vi "Parse PROCAR.vi"(10 "Extract Decomposed Band?":bool, 11 "Path":path) -> (0 "KS Bandgap (eV)":dbl, 1 "CBM Band Index":i32, 2 "Decomposed Band Structure":T1(array[cluster]), 3 "Band Structure":T2(array[cluster]))   [LabVIEW 2010]
uses:
  <vilib>/Utility/error.llb/DialogType.ctl
  <vilib>/Analysis/_algsub.llb/Real Vector Norm.vi
  <vilib>/Analysis/NI_AALPro.lvlib
panel:
  out "CBM (eV)":dbl
  out "VBM (eV)":dbl
  in  "balance parameter":dbl=-1.0
  in  "# of points per slope":i16=4
  out "System XY Graph 3":cluster{i32[], "dY/dX":dbl[]}[](graph)
  out "1st Deriv":cluster{i32[], "Best Cubic Spline Fit":dbl[]}[](graph)
  out "Calc time (ms)":u32
  in  "Bands to Plot":i32[](array[numeric])
  out "System XY Graph":cluster{i32[], dbl[]}[](graph)
  out "# of Ions":i32
  out "# of Bands":i32
  out "# k points":i32
  # "Gamma"
  # "X"
  # "L"
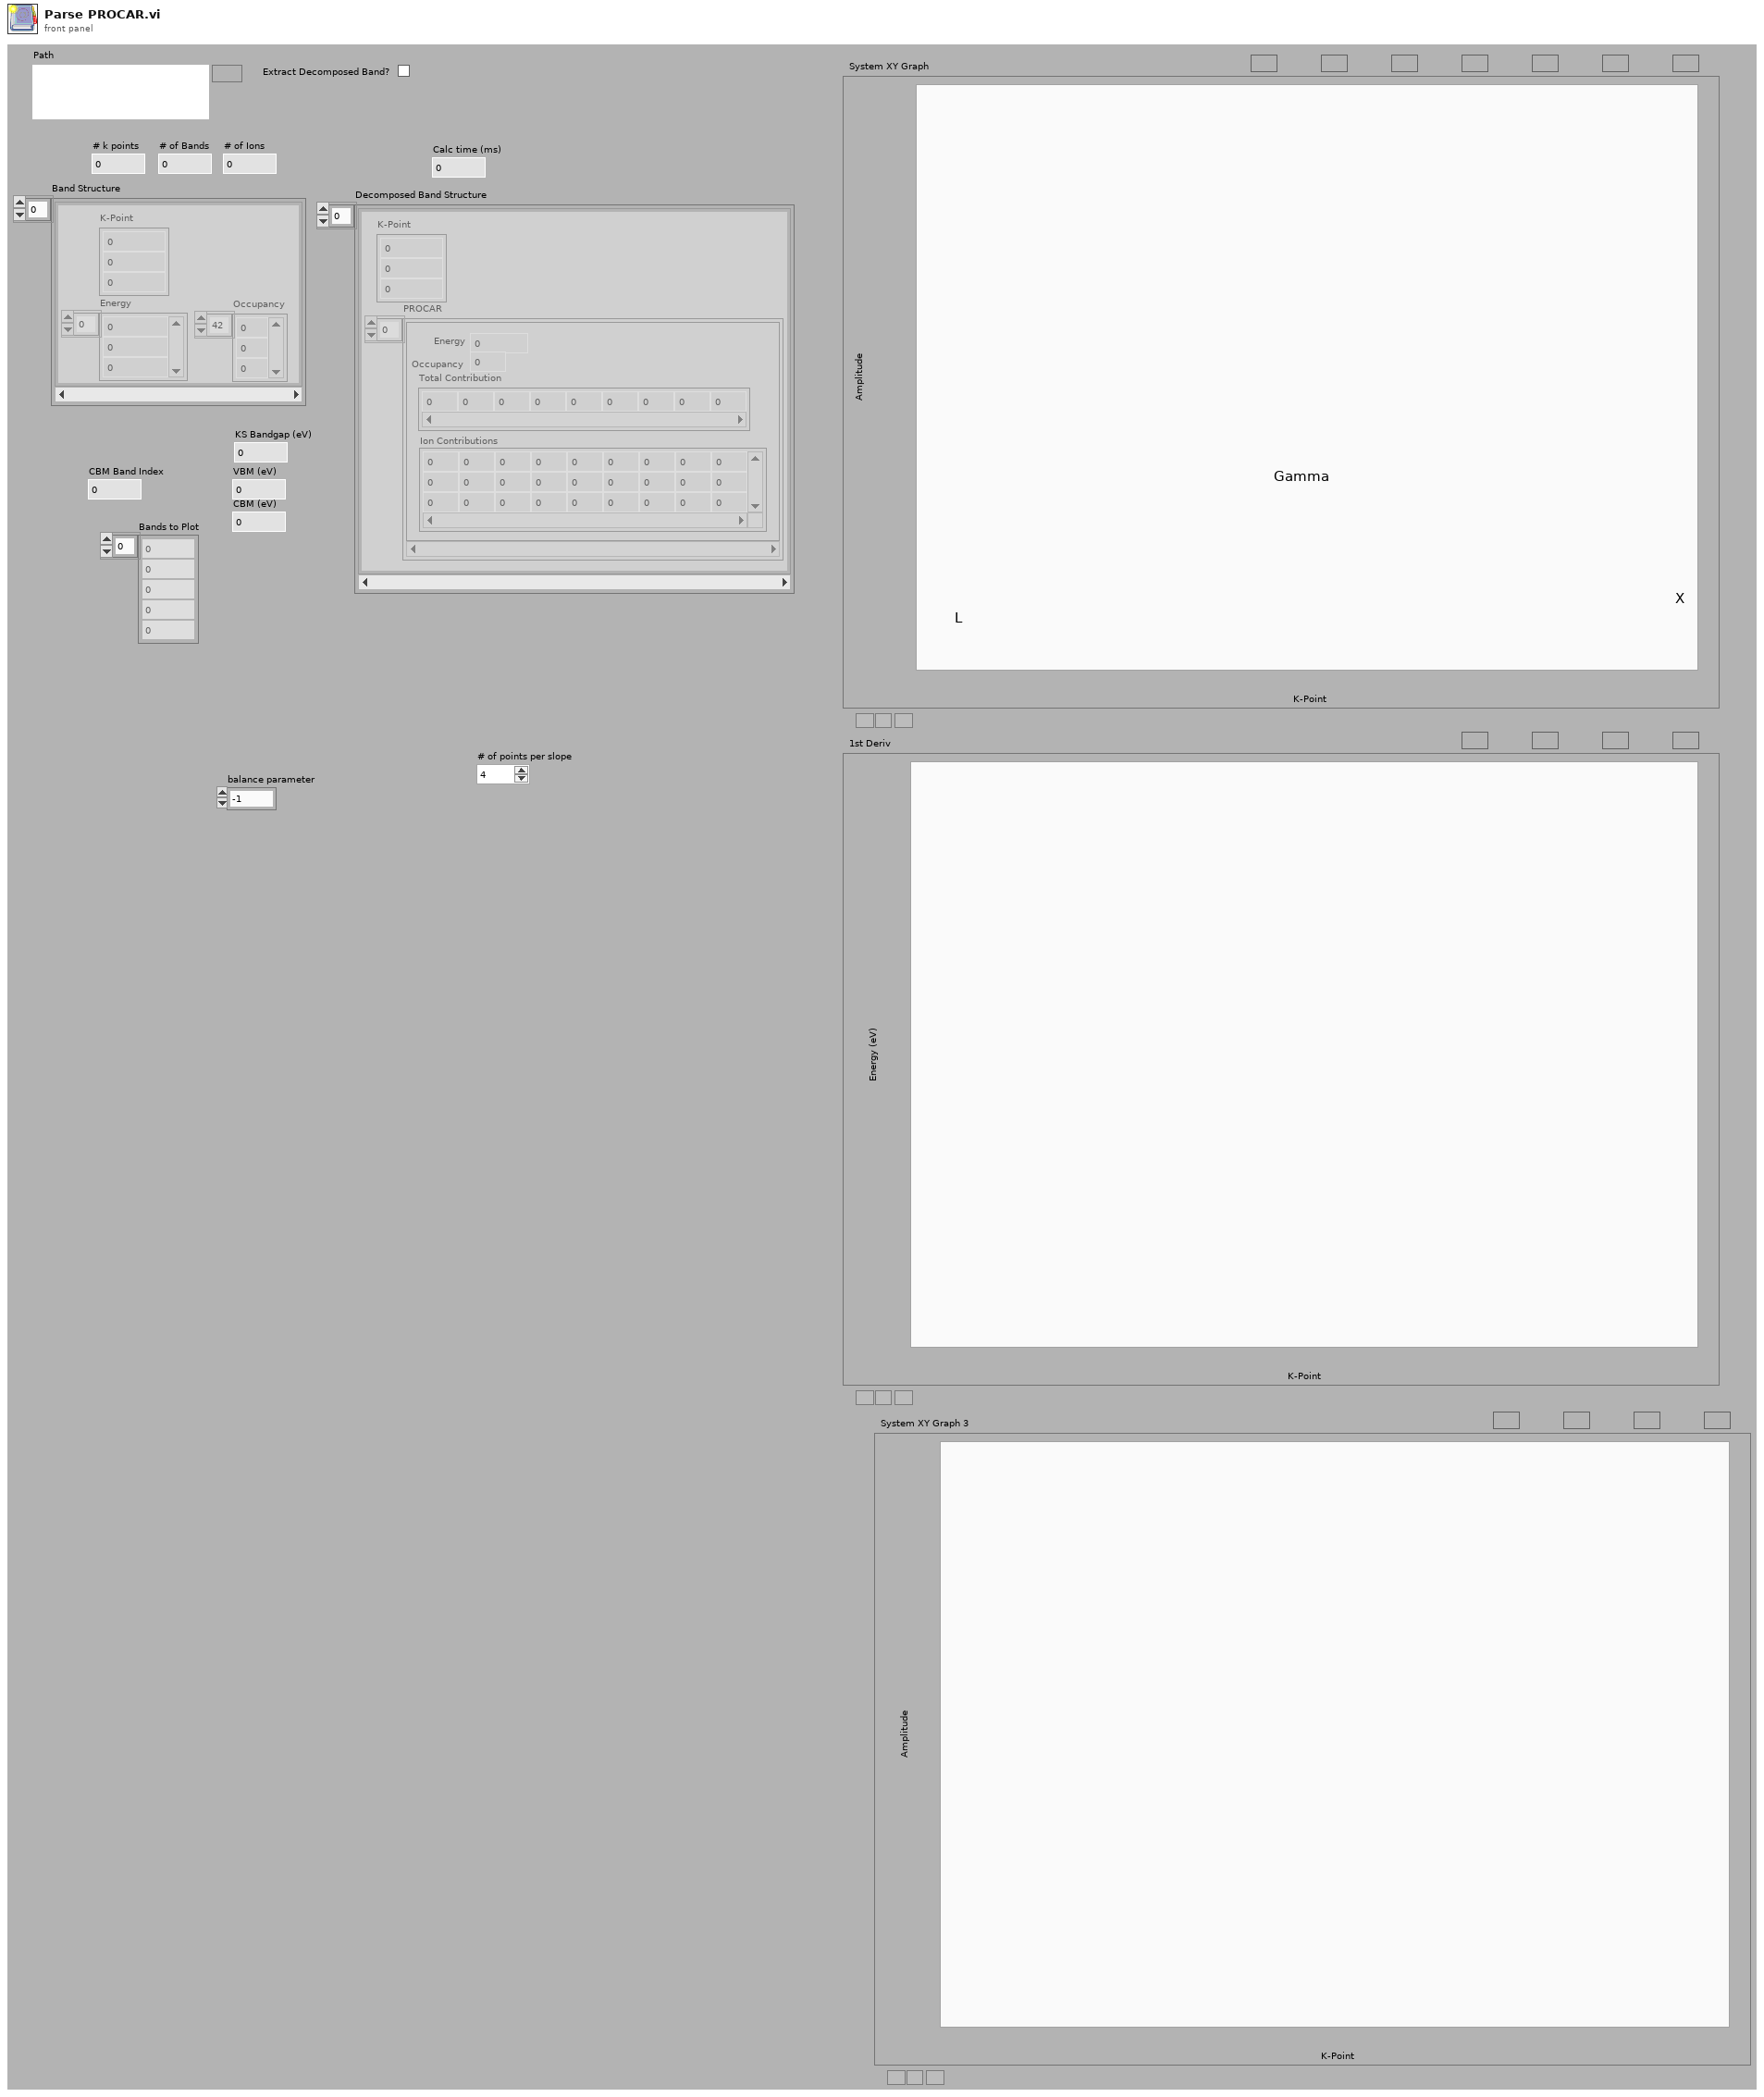
[diagram p1: front panel]
types:
  T1 = cluster{"K-Point":dbl[], "PROCAR":cluster{"Energy":dbl, "Occupancy":dbl, "Total Contribution":dbl[], "Ion Contributions":dbl[][]}[]}[]
  T2 = cluster{"K-Point":dbl[], "Energy":dbl[], "Occupancy":dbl[]}[]
  T3 = cluster{"number 3":dbl[], cluster{dbl, dbl, dbl[], dbl[][]}[]}[]
  T4 = cluster{"number 3":dbl[], "number 3":dbl[], "number 3":dbl[]}
  T5 = cluster{"number 3":dbl[], cluster{dbl, dbl, dbl[], dbl[][]}[]}
  T6 = cluster{"number 3":dbl[], "number 3":dbl[], "number 3":dbl[]}[]
  T7 = typedef "DialogType.ctl" = u16
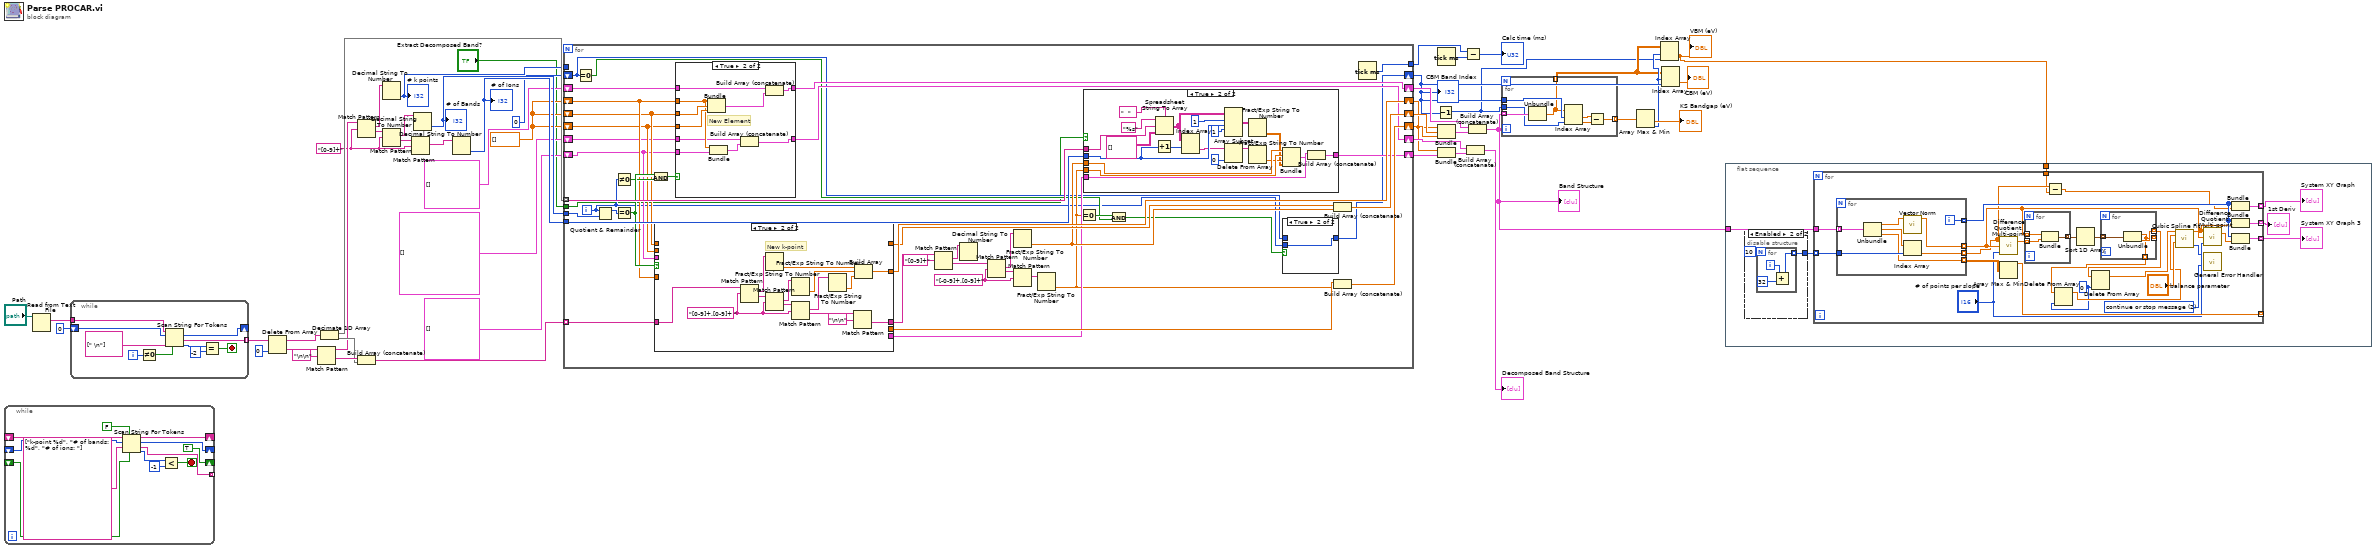
[diagram p0: block diagram]
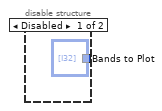
[diagram p2: hidden frame]
diagram:
  w27 = dbl[] [] ("number 3")
  w34 = "[0-9]+"
  n1 = while {
    shift-right: [w59] -> _
    shift-left: _ -> [w60]
    tunnel: [w58] -> _ mode=indexing
    shift-right: [w57] -> _
    shift-left: _ -> [w56]
    shift-right: [TRUE ("allow empty tokens? (F)")] -> _
    shift-left: _ -> [w52]
    stop <- w53 stop-if-true
    n2 = Scan String For Tokens(4:w52, 5:FALSE ("allow empty tokens? (F)"), 7:string[] ["k-point %d", "# of bands: %d", "# of ions: "] ("operators (none)"), 8:w56, 9:w60) -> (0:w55:i32, 1:w58:string, 2:w57:i32, 3:w59:string)  [unwired: 1 in]
    n3 = Less?(x=w55, y=-1) -> (x < y?=w53:bool)
  }
  n4 = Read from Text File(file (use dialog)="Path") -> (text=w48:string)  [unwired: 3 in, 3 out]
  n5 = while {
    tunnel: w48 -> [w71]
    shift-right: [w63] -> _
    shift-left: 0 ("offset past token") -> [w62]
    tunnel: [w70] -> w46 mode=indexing
    i -> [w68]
    stop <- w64 stop-if-true
    n6 = Not Equal To 0?(x=w68) -> (x != 0?=w67:bool)
    n7 = Scan String For Tokens(4:w67, 6:string[] [" \n"] ("delimiters (\\s,\\t,\\r,\\n)"), 8:w62, 9:w71) -> (0:w66:i32, 1:w70:string, 2:w63:i32)  [unwired: 2 in, 1 out]
    n8 = Equal?(x=w66, y=-2) -> (x = y?=w64:bool)
  }
  n9 = Delete From Array(array=w46, index=0) -> (deleted portion=w44:string, array with subset deleted=w45:string[])  [unwired: 1 in]
  n10 = Match Pattern(string=w44, regular expression="\n\n") -> (before substring=w37:string, after substring=w42:string)  [unwired: 1 in, 2 out]
  n11 = Decimate 1D Array(w45) -> (w38:string[], w41:string[])
  n12 = Match Pattern(string=w37, regular expression=w34) -> (match substring=w33:string, after substring=w36:string)  [unwired: 1 in, 2 out]
  n13 = Build Array (concatenate)(w42, w41) -> (w39:string[])
  n14 = Decimal String To Number(string=w33) -> (number=w26:i32)  [unwired: 2 in, 1 out]
  "# k points" <- w26
  n15 = Match Pattern(string=w36, regular expression=w34) -> (match substring=w32:string, after substring=w35:string)  [unwired: 1 in, 2 out]
  n16 = Match Pattern(string=w35, regular expression=w34) -> (match substring=w31:string)  [unwired: 1 in, 3 out]
  n17 = Decimal String To Number(string=w32) -> (number=w29:i32)  [unwired: 2 in, 1 out]
  "# of Bands" <- w29
  n18 = Decimal String To Number(string=w31) -> (number=w30:i32)  [unwired: 2 in, 1 out]
  "# of Ions" <- w30
  n19 = for {
    tunnel: w38 -> [w112] mode=indexing
    tunnel: w39 -> [w103] mode=indexing
    tunnel: w30 -> [w111]
    tunnel: w29 -> [w93]
    shift-right: [w104] -> w18
    shift-left: w27 -> [w92]
    shift-right: [w88] -> w23
    shift-left: T2 [] ("Band Structure") -> [w89]
    shift-right: [w98] -> w25
    shift-left: w27 -> [w91]
    shift-right: [w99] -> w24
    shift-left: w27 -> [w90]
    tunnel: w26 -> [_]
    shift-right: [w85] -> w17
    shift-left: cluster{dbl, dbl, dbl[], dbl[][]}[] [] -> [w82]
    shift-right: [w84] -> w19
    shift-left: T3 [] -> [w83]
    shift-right: [w76] -> w6
    shift-left: 0 ("# of Ions 2") -> [w74]
    tunnel: [w73] -> w8
    tunnel: "Extract Decomposed Band?" -> [w72]
    i -> [w75]
    w105 = "[-0-9]+.[0-9]+" ("regular expression")
    n20 = Equal To 0?(x=w74) -> (x = 0?=w78:bool)
    n21 = Quotient & Remainder(x=w75, y=w93) -> (x-y*floor(x/y)=w102:i32)  [unwired: 1 out]
    n22 = Not Equal To 0?(x=w75) -> (x != 0?=w94:bool)
    n23 = Equal To 0?(x=w102) -> (x = 0?=w95:bool)
    n24 = And(x=w95, y=w94) -> (x .and. y?=w87:bool)
    n25 = case shown="True" w95 {
      tunnel: w103 -> [w151 w165]
      tunnel: w92 -> [w150 _]
      tunnel: [w150 w152] -> w104
      tunnel: [w151 w164] -> w106
      tunnel: w91 -> [w149 _]
      tunnel: w90 -> [w148 _]
      tunnel: [w149 _] -> w97
      tunnel: [w148 _] -> w96
      tunnel: w82 -> [w147 _]
      tunnel: [w147 _] -> w81
      frame False {
        # "Only new band"
      }
      frame True {
        w161 = "[0-9]+.[0-9]+ " ("regular expression")
        # "New k-point"
        n26 = Match Pattern(string=w165, regular expression=w161) -> (match substring=w155:string, after substring=w163:string)  [unwired: 1 in, 2 out]
        n27 = Fract/Exp String To Number(string=w155) -> (number=w159:dbl)  [unwired: 3 in, 1 out]
        n28 = Match Pattern(string=w163, regular expression=w161) -> (match substring=w160:string, after substring=w162:string)  [unwired: 1 in, 2 out]
        n29 = Fract/Exp String To Number(string=w160) -> (number=w158:dbl)  [unwired: 3 in, 1 out]
        n30 = Match Pattern(string=w162, regular expression=w161) -> (match substring=w156:string, after substring=w154:string)  [unwired: 1 in, 2 out]
        n31 = Fract/Exp String To Number(string=w156) -> (number=w157:dbl)  [unwired: 3 in, 1 out]
        n32 = Match Pattern(string=w154, regular expression="\n\n") -> (after substring=w164:string)  [unwired: 1 in, 3 out]
        n33 = Build Array(w159, w158, w157) -> (w152:dbl[])
      }
    }
    n34 = case shown="True" w87 {
      tunnel: w92 -> [_ w141]
      tunnel: w91 -> [_ w146]
      tunnel: w90 -> [_ w145]
      tunnel: w89 -> [w136 w144]
      tunnel: [w136 w143] -> w88
      tunnel: w82 -> [_ w142]
      tunnel: [w135 w139] -> w84
      tunnel: w83 -> [w135 w138]
      frame False {
      }
      frame True {
        # "New Element"
        n35 = Bundle("number 3"=w141, "number 3"=w146, "number 3"=w145) -> (w137:T4)  [unwired: 1 in]
        n36 = Bundle("number 3"=w141, w142) -> (w140:T5)  [unwired: 1 in]
        n37 = Build Array (concatenate)(w138, w140) -> (w139:T3)
        n38 = Build Array (concatenate)(w144, w137) -> (w143:T6)
      }
    }
    n39 = Match Pattern(string=w106, regular expression="[0-9]+") -> (match substring=w107:string, after substring=w110:string)  [unwired: 1 in, 2 out]
    n40 = Decimal String To Number(string=w107) -> ()  [unwired: 2 in, 2 out]
    n41 = Match Pattern(string=w110, regular expression=w105) -> (match substring=w101:string, after substring=w109:string)  [unwired: 1 in, 2 out]
    n42 = Fract/Exp String To Number(string=w101) -> (number=w86:dbl)  [unwired: 3 in, 1 out]
    n43 = Match Pattern(string=w109, regular expression=w105) -> (match substring=w100:string)  [unwired: 1 in, 3 out]
    n44 = Fract/Exp String To Number(string=w100) -> (number=w80:dbl)  [unwired: 3 in, 1 out]
    n45 = Equal To 0?(x=w80) -> (x = 0?=w79:bool)
    n46 = case shown="True" w72 {
      tunnel: w112 -> [_ w132]
      tunnel: w111 -> [_ w131]
      tunnel: w86 -> [_ w130]
      tunnel: [_ w129] -> w85
      tunnel: w81 -> [_ w128]
      tunnel: w80 -> [_ w127]
      frame False {
      }
      frame True {
        n47 = Increment(x=w131) -> (x+1=w119:i32)
        n48 = Spreadsheet String To Array(delimiter (Tab)="  ", format string="%s", spreadsheet string=w132, array type (2D Dbl)=string[][] []) -> (array=w120:string[][])
        n49 = Index Array(array=w120, index (row)=w119) -> (element=w118:string[])  [unwired: 1 in]
        n50 = Array Subset(array=w120, index (row)=1 ("index"), length (row)=w131, index (col)=1 ("index")) -> (w115:string[][])  [unwired: 1 in]
        n51 = Delete From Array(array=w118, index=0) -> (array with subset deleted=w116:string[])  [unwired: 1 in, 1 out]
        n52 = Fract/Exp String To Number(string=w115) -> (number=w113:dbl[][])  [unwired: 3 in, 1 out]
        n53 = Fract/Exp String To Number(string=w116) -> (number=w114:dbl[])  [unwired: 3 in, 1 out]
        n54 = Bundle(w130, w127, w114, w113) -> (w126:cluster{dbl, dbl, dbl[], dbl[][]})  [unwired: 1 in]
        n55 = Build Array (concatenate)(w128, w126) -> (w129:cluster{dbl, dbl, dbl[], dbl[][]}[])
      }
    }
    n56 = And(x=w79, y=w78) -> (x .and. y?=w77:bool)
    n57 = case shown="True" w77 {
      tunnel: [w133 w134] -> w76
      tunnel: w75 -> [_ w134]
      tunnel: w74 -> [w133 _]
      frame False {
      }
      frame True {
      }
    }
    n58 = Build Array (concatenate)(w97, w86) -> (w98:dbl[])
    n59 = Build Array (concatenate)(w96, w80) -> (w99:dbl[])
    n60 = Tick Count (ms)() -> (millisecond timer value=w73:u32)
  }
  "CBM Band Index" <- w6
  n61 = Decrement(x=w6) -> (x-1=w3:i32)
  n62 = Tick Count (ms)() -> (millisecond timer value=w12:u32)
  n63 = Bundle("number 3"=w18, "number 3"=w25, "number 3"=w24) -> (w22:T4)  [unwired: 1 in]
  n64 = Bundle("number 3"=w18, w17) -> (w16:T5)  [unwired: 1 in]
  n65 = Subtract(x=w8, y=w12) -> (x-y=→"Calc time (ms)":u32)
  n66 = Build Array (concatenate)(w19, w16) -> (→"Decomposed Band Structure":T3)
  n67 = Build Array (concatenate)(w23, w22) -> (w13:T6)
  "Band Structure" <- w13
  n68 = for {
    tunnel: w13 -> [w172] mode=indexing
    tunnel: w3 -> [w170]
    tunnel: w6 -> [w171]
    tunnel: [w167] -> w10 mode=indexing
    tunnel: [w166] -> w4 mode=indexing
    n69 = Unbundle(w172) -> ("number 3"=w166:dbl[])  [unwired: 2 out]
    n70 = Index Array(array=w166, index #1=w171, index #2=w170) -> (element #1=w169:dbl, element #2=w168:dbl)
    n71 = Subtract(x=w169, y=w168) -> (x-y=w167:dbl)
  }
  n72 = Array Max & Min(array=w10) -> (min value=→"KS Bandgap (eV)":dbl, min index (indices)=w5:i32)  [unwired: 2 out]
  n73 = Index Array(array=w4, index (row)=w5, index (col)=w3) -> (element=w1:dbl)
  "VBM (eV)" <- w1
  n74 = Index Array(array=w4, index (row)=w5, index (col)=w6) -> (element=→"CBM (eV)":dbl)
  n75 = flat-sequence {
    tunnel: w13 -> [w178]
    tunnel: w1 -> [w173]
    frame #0 {
      n76 = disable-structure shown="Enabled" {
        disable-tunnel: ["Bands to Plot" w181] -> w177
        frame Disabled {
        }
        frame Enabled {
          n77 = for {
            N: 10 -> [_]
            tunnel: [w183] -> w181 mode=indexing
            i -> [w184]
            n78 = Add(x=w184, y=32) -> (x+y=w183:i32)
          }
        }
      }
      n79 = for {
        tunnel: w178 -> [w209]
        tunnel: w177 -> [w210] mode=indexing
        tunnel: [w208] -> w176 mode=indexing
        tunnel: [w206] -> _ mode=indexing
        tunnel: [w205] -> w175 mode=indexing
        tunnel: [w203] -> w174 mode=indexing
        tunnel: w173 -> [w186]
        w188 = 0 ("index")
        w193 = T7 2 items=["no dialog", "OK message", "continue or stop message", "OK message + warnings", "continue/stop + warnings"] ("type of dialog (OK msg:1)")
        n80 = for {
          tunnel: w210 -> [w222]
          tunnel: w209 -> [w224] mode=indexing
          tunnel: [w221] -> w187 mode=indexing
          tunnel: [w220] -> w201 mode=indexing
          tunnel: [w219] -> w207 mode=indexing
          tunnel: [w217] -> w197 mode=indexing
          i -> [w220]
          n81 = Unbundle(w224) -> ("number 3"=w218:dbl[], "number 3"=w223:dbl[], "number 3"=w219:dbl[])
          n82 = call-poly <vilib>:"Vector Norm.vi"("Input Vector"=w218) -> ("norm"=w217:dbl)  [unwired: 9 in, 1 out]
          n83 = Index Array(array=w223, index=w222) -> (element=w221:dbl)
        }
        n84 = call "Difference Quotient, Multi-point.vi"("# of points per slope"="# of points per slope", "X"=w197, "Y"=w187) -> ("dY/dX"=w200:dbl[])  [unwired: 1 in]
        n85 = Array Max & Min(array=w207) -> (max value=w206:dbl)  [unwired: 3 out]
        n86 = for {
          tunnel: w197 -> [w215] mode=indexing
          tunnel: w200 -> [w216] mode=indexing
          tunnel: [w214] -> w199 mode=indexing
          n87 = Bundle("norm"=w215, w216) -> (w214:cluster{"norm":dbl, dbl})  [unwired: 1 in]
        }
        n88 = Subtract(x=w187, y=w186) -> (x-y=w185:dbl[])
        n89 = Sort 1D Array(array=w199) -> (sorted array=w198:cluster{"norm":dbl, dbl}[])
        n90 = for {
          tunnel: w198 -> [w213] mode=indexing
          tunnel: [w211] -> _ mode=indexing
          tunnel: [w212] -> w192 mode=indexing
          tunnel: [w211] -> w190 mode=indexing
          n91 = Unbundle(w213) -> ("norm"=w211:dbl, w212:dbl)
        }
        n92 = Delete From Array(array=w190, index=w188) -> (array with subset deleted=w189:dbl[])  [unwired: 1 in, 1 out]
        n93 = Delete From Array(array=w192, index=w188) -> (array with subset deleted=w191:dbl[])  [unwired: 1 in, 1 out]
        n94 = call <vilib>:"Cubic Spline Fit.vi"("Y"=w191, "X"=w189, "balance parameter"="balance parameter") -> ("Best Cubic Spline Fit"=w196:dbl[], "error"=w194:i32)  [unwired: 11 in]
        n95 = call "Difference Quotient, Multi-point.vi"("# of points per slope"="# of points per slope", "X"=w197, "Y"=w196) -> ("dY/dX"=w204:dbl[])  [unwired: 1 in]
        n96 = call <vilib>:"General Error Handler.vi"("[error code] (0)"=w194, "type of dialog (OK msg:1)"=w193) -> ()  [unwired: 9 in, 5 out]
        n97 = Bundle(w201, w185) -> (w208:cluster{i32[], dbl[]})  [unwired: 1 in]
        n98 = Bundle(w201, "Best Cubic Spline Fit"=w196) -> (w205:cluster{i32[], "Best Cubic Spline Fit":dbl[]})  [unwired: 1 in]
        n99 = Bundle(w201, "dY/dX"=w204) -> (w203:cluster{i32[], "dY/dX":dbl[]})  [unwired: 1 in]
      }
      "System XY Graph" <- w176
      "1st Deriv" <- w175
      "System XY Graph 3" <- w174
    }
  }
